vi "Create E&S Text file.vi"(0 "file path (use dialog)":path, 11 "error in (no error)":errorcluster, 12 "Simple(F)":bool) -> (4 "refnum out":refnum<file>, 15 "error out":errorcluster)   [LabVIEW 2011]
uses:
  <vilib>/Utility/libraryn.llb/Check if File or Folder Exists.vi
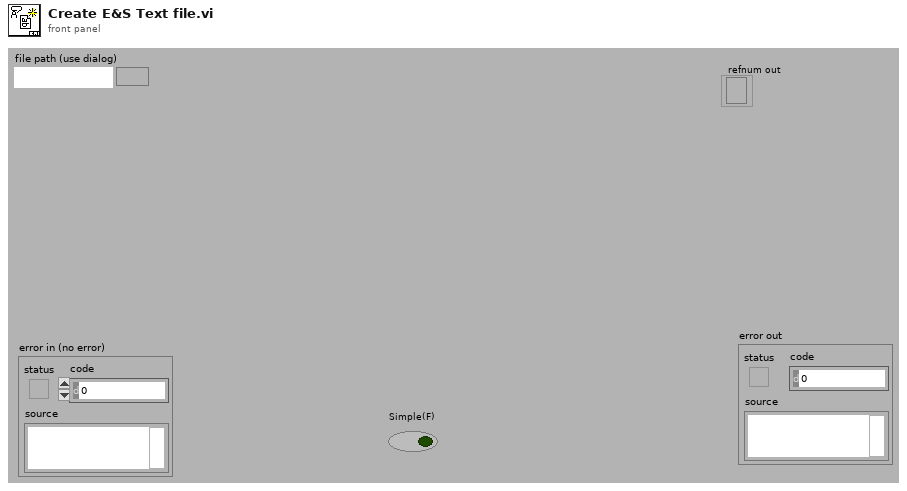
[diagram p1: front panel]
types:
  T1 = enum16{"open", "replace", "create", "open or create", "replace or create", "replace or create with confirmation"}
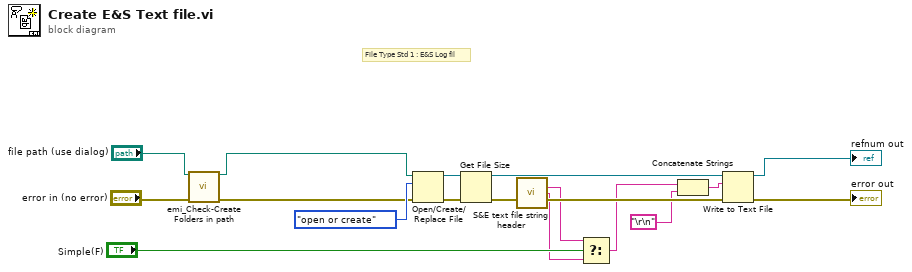
[diagram p0: block diagram]
diagram:
  # "File Type Std 1 : E&S Log fil"
  n1 = call "emi_Check-Create Folders in path.vi"("Path including file"="file path (use dialog)", "error in (no error)"="error in (no error)") -> ("Path out"=w1:path, "error out"=w3:errorcluster)  [unwired: 11 in, 1 out]
  n2 = Open/Create/Replace File(file path (use dialog)=w1, error in=w3, operation (0:open)=T1."open or create") -> (refnum out=w16:refnum<file>, error out=w17:errorcluster)  [unwired: 3 in, 1 out]
  n3 = Get File Size(file=w16, error in=w17) -> (refnum out=w11:refnum<file>, 0:w12:errorcluster)  [unwired: 1 out]
  n4 = call "S&E text file string header.vi"("error in (no error)"=w12) -> ("Simple Header"=w9:string, "Full Header"=w8:string, "error out"=w15:errorcluster)  [unwired: 12 in]
  n5 = Select(t=w9, s="Simple(F)", f=w8) -> (s? t:f=w7:string)
  n6 = Concatenate Strings(w7, "\r\n") -> (w14:string)
  n7 = Write to Text File(file (use dialog)=w11, text=w14, error in=w15) -> (refnum out=→"refnum out":refnum<file>, error out=→"error out":errorcluster)  [unwired: 1 in, 1 out]
